vi "Page_Exclusions_Initialize.vi"(8 "error in (no error)":errorcluster, 9 "ctlReferences":T1, 11 "AB_Application in":refnum<class "AB_Application.lvclass">) -> (0 "error out":errorcluster, 3 "AB_Application out":refnum<class "AB_Application.lvclass">)   [LabVIEW 2020, in "AB_Application.lvclass"]
uses:
  <vilib>/AppBuilder/AB_Classes/Application/AB_Application.lvclass
  <resource>/Framework/Providers/Builds/AppBuilder/AB_UI_Page_Exclusions_References.ctl
  <vilib>/AppBuilder/AB_Classes/TargetFile/AB_Targetfile.lvclass
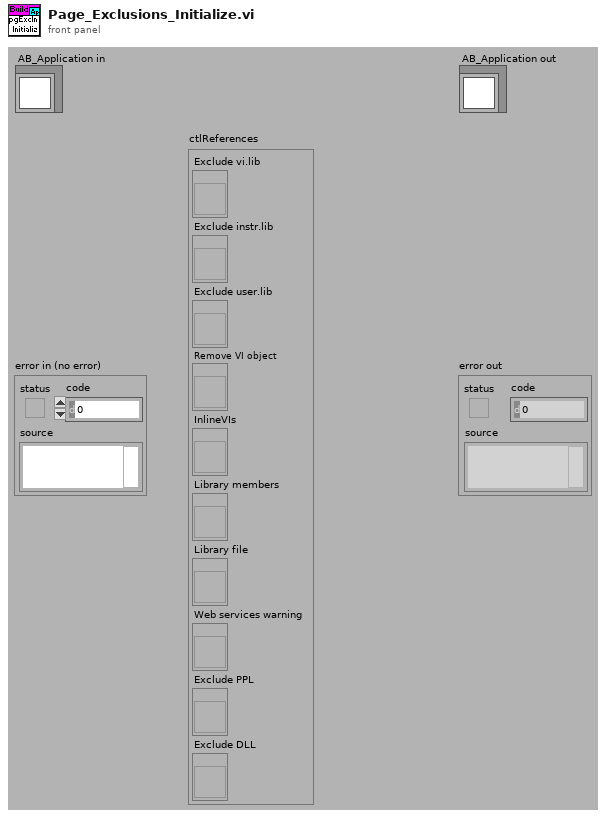
[diagram p1: front panel]
types:
  T1 = typedef "AB_UI_Page_Exclusions_References.ctl" = cluster{"Exclude vi.lib":refnum<vi>, "Exclude instr.lib":refnum<vi>, "Exclude user.lib":refnum<vi>, "Remove VI object":refnum<vi>, "InlineVIs":refnum<vi>, "Library members":refnum<vi>, "Library file":refnum<vi>, "Web services warning":refnum<vi>, "Exclude PPL":refnum<vi>, "Exclude DLL":refnum<vi>}
  T2 = typedef "LVPositionTypeDef.ctl" = cluster{"Left":i32, "Top":i32}
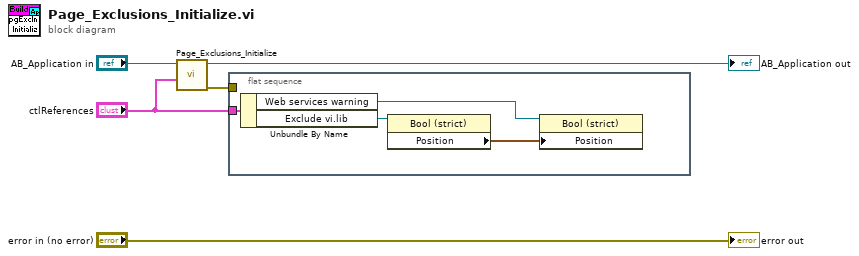
[diagram p0: block diagram]
diagram:
  n1 = call-parent "Page_Exclusions_Initialize.vi"("ctlReferences"="ctlReferences", "AB_Targetfile in"="AB_Application in") -> ("error out"=w2:errorcluster, "AB_Targetfile out"=→"AB_Application out":refnum<class "AB_Application.lvclass">)  [unwired: 8 in]
  n2 = flat-sequence {
    tunnel: "ctlReferences" -> [w6]
    tunnel: w2 -> [_]
    frame #0 {
      n3 = Unbundle By Name(w6) -> ("Web services warning"=w9:refnum<vi>, "Exclude vi.lib"=w8:refnum<vi>)
      n4 = property class="Bool (strict)"(reference=w8) -> ("Position"=w7:T2)  [unwired: 1 in, 2 out]
      n5 = property class="Bool (strict)"(reference=w9, "Position"=w7) -> ()  [unwired: 1 in, 2 out]
    }
  }
  "error out" <- "error in (no error)"
